vi "Read Dev Parameters.vi"(8 "error in (no error)":errorcluster, 11 "VISA resource name":refnum<visa-resource-name>) -> (0 "error out":errorcluster, 2 "dev parameters":T1, 3 "VISA resource name out":refnum<visa-resource-name>)   [LabVIEW 2020, in "Andeen-Hagerling 2700A.lvlib"]
doc: "Read the deviation parameters which may vary with other analog out or deviation paramters. Includes dev point, dev position, dev bounds, and dev span."
uses:
  Andeen-Hagerling 2700A.lvlib
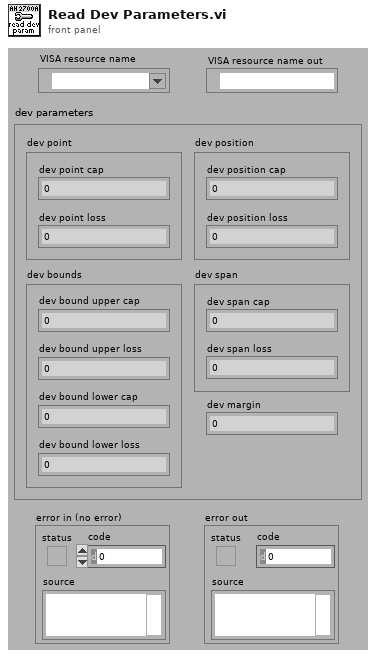
[diagram p1: front panel]
types:
  T1 = cluster{"dev bounds":cluster{"dev bound upper cap":dbl, "dev bound upper loss":dbl, "dev bound lower cap":dbl, "dev bound lower loss":dbl}, "dev point":cluster{"dev point cap":dbl, "dev point loss":dbl}, "dev position":cluster{"dev position cap":dbl, "dev position loss":dbl}, "dev span":cluster{"dev span cap":dbl, "dev span loss":dbl}, "dev margin":dbl}
  T2 = cluster{"dev bound upper cap":dbl, "dev bound upper loss":dbl, "dev bound lower cap":dbl, "dev bound lower loss":dbl}
  T3 = cluster{"dev point cap":dbl, "dev point loss":dbl}
  T4 = cluster{"dev position cap":dbl, "dev position loss":dbl}
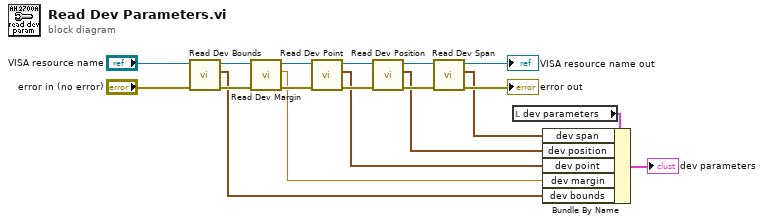
[diagram p0: block diagram]
diagram:
  n1 = call "Read Dev Bounds.vi"("error in (no error)"="error in (no error)", "VISA resource name"="VISA resource name") -> ("error out"=w11:errorcluster, "dev bounds"=w2:T2, "VISA resource name out"=w15:refnum<visa-resource-name>)  [unwired: 7 in]
  n2 = call "Read Dev Margin.vi"("error in (no error)"=w11, "VISA resource name"=w15) -> ("error out"=w10:errorcluster, "dev margin"=w3:dbl, "VISA resource name out"=w14:refnum<visa-resource-name>)  [unwired: 7 in]
  n3 = call "Read Dev Point.vi"("error in (no error)"=w10, "VISA resource name"=w14) -> ("error out"=w9:errorcluster, "dev point"=w4:T3, "VISA resource name out"=w13:refnum<visa-resource-name>)  [unwired: 7 in]
  n4 = call "Read Dev Position.vi"("error in (no error)"=w9, "VISA resource name"=w13) -> ("error out"=w8:errorcluster, "dev position"=w5:T4, "VISA resource name out"=w12:refnum<visa-resource-name>)  [unwired: 7 in]
  n5 = call "Read Dev Span.vi"("error in (no error)"=w8, "VISA resource name"=w12) -> ("error out"=→"error out":errorcluster, "dev span"=w6:cluster{"dev span cap":dbl, "dev span loss":dbl}, "VISA resource name out"=→"VISA resource name out":refnum<visa-resource-name>)  [unwired: 7 in]
  n6 = local read "dev parameters"() -> (w7:T1)
  n7 = Bundle By Name(cluster=w7, "dev span"=w6, "dev position"=w5, "dev point"=w4, "dev margin"=w3, "dev bounds"=w2) -> (→"dev parameters":T1)
